vi "New Digital Writer.vi"(8 "error in (no error)":errorcluster, 10 "DAQmx Task":refnum<k21>, 11 "Digital Writer in":refnum<class "Digital Writer.lvclass">) -> (0 "error out":errorcluster, 3 "Digital Writer out":refnum<class "Digital Writer.lvclass">)   [LabVIEW 2024, in "DAQmx Actor.lvlib" / "Digital Writer.lvclass"]
uses:
  Digital Writer.lvclass
  Digital Writer.lvclass/Digital Writer.ctl
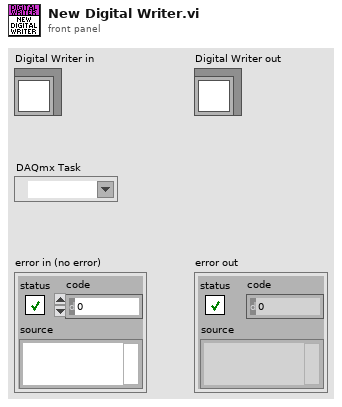
[diagram p1: front panel]
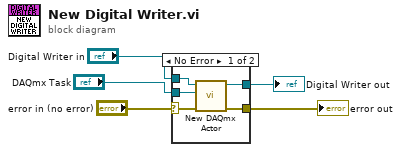
[diagram p0: block diagram]
diagram:
  n1 = case shown="No Error" "error in (no error)" {
    selector: "error in (no error)" -> [w8 w12]
    tunnel: [w7 w12] -> w4
    tunnel: [w6 w11] -> w2
    tunnel: "Digital Writer in" -> [w10 w11]
    tunnel: "DAQmx Task" -> [w9 _]
    frame No Error {
      n2 = call-dynamic "New DAQmx Actor.vi"("error in (no error)"=w8, "DAQmx Task"=w9, "DAQmx Actor in"=w10) -> ("error out"=w7:errorcluster, "DAQmx Actor out"=w6:refnum<class "Digital Writer.lvclass">)  [unwired: 7 in]
    }
    frame Error {
    }
  }
  "error out" <- w4
  "Digital Writer out" <- w2
